vi "Push Points Batch.vi"   [LabVIEW 2020, in "Nominal Streaming.lvlib" / "Channel.lvclass"]
doc: "Pushes point data to Nominal Core.\nData can be presented in either [{timestamp, value}] or [{value, timestamp}].\nAny `Not a Number` (NaN) values will be filtered out.\nReturns an error if there is a mismatch in input array sizes."
uses:
  Channel.lvclass
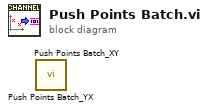
[diagram p0: block diagram]
diagram:
  n1 = call "Push Points Batch_YX.vi"() -> ()  [unwired: 10 in, 2 out]
  n2 = call "Push Points Batch_XY.vi"() -> ()  [unwired: 10 in, 2 out]
